vi "SettingsText.vi"(8 "Saved code":string, 10 "Python Code in":string, 11 "VI in":refnum<vi>) -> (2 "Python Code out":string, 3 "VI out":refnum<vi>)   [LabVIEW 2017]
panel:
  in  "Blob Params":T1={"Feature"=5, "Lab thresholds"="[10,90,-20,20,-20,20]", "Minimum Pixels"=100, "Minimum Area (box)"=100, "Merge"=TRUE, "Margin for merge"=10} {"Feature" items=["x", "y", "width", "height", "pixels", "cx", "cy", "rotation", "code", "count", "# blobs", "All parameters"]}
  in  "WiFi Info":T2
  in  "ROI":T3
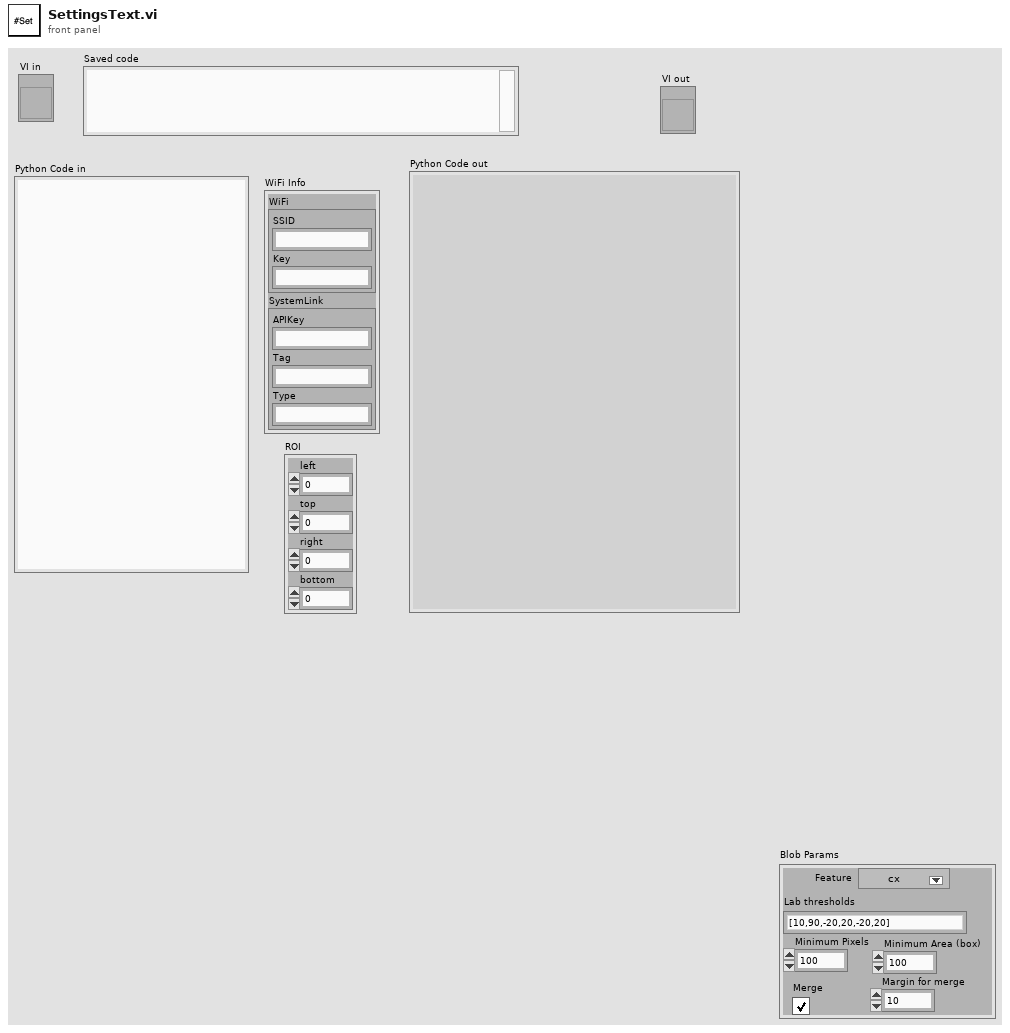
[diagram p1: front panel]
types:
  T1 = cluster{"Feature":u16, "Lab thresholds":string, "Minimum Pixels":i16, "Minimum Area (box)":i16, "Merge":bool, "Margin for merge":i16}
  T2 = cluster{"WiFi":cluster{"SSID":string, "Key":string}, "SystemLink":cluster{"APIKey":string, "Tag":string, "Type":string}}
  T3 = cluster{"left":i32, "top":i32, "right":i32, "bottom":i32}
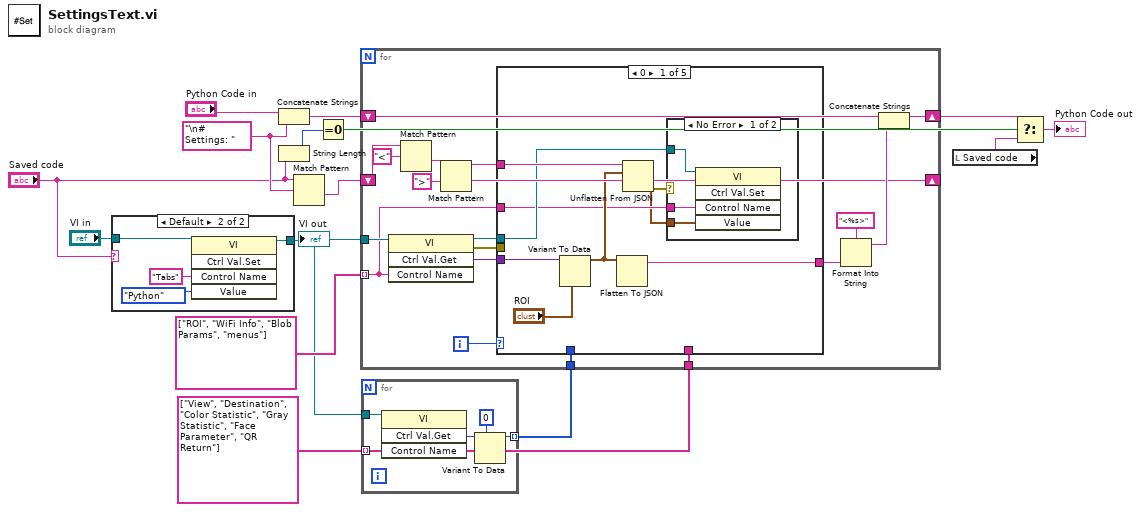
[diagram p0: block diagram]
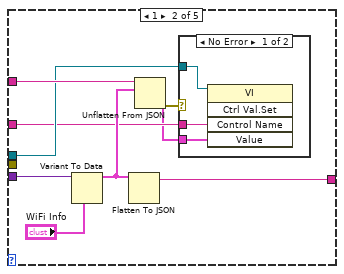
[diagram p4: hidden frame]
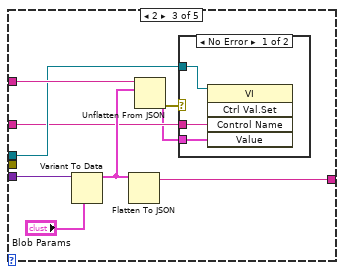
[diagram p6: hidden frame]
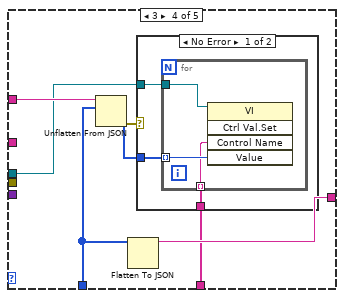
[diagram p8: hidden frame]
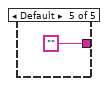
[diagram p10: hidden frame]
diagram:
  w9 = string[] ["View", "Destination", "Color Statistic", "Gray Statistic", "Face Parameter", "QR Return"]
  w11 = "\n# Settings: " ("string")
  n1 = case shown="Default" "Saved code" {
    tunnel: "VI in" -> [w16 w19]
    tunnel: [w16 w18] -> w2
    frame "\u0000" {
    }
    frame Default {
      n2 = invoke class="VI" method="Ctrl Val.Set"(reference=w19, "Control Name"="Tabs", "Value"=enum32{"Simple View", "REPL", "Python"}."Python" ("Tabs")) -> (reference out=w18:refnum<vi>)  [unwired: 2 in, 4 out]
    }
  }
  "VI out" <- w2
  n3 = Concatenate Strings("Python Code in", w11) -> (w13:string)
  n4 = String Length(string="Saved code") -> (length=w6:i32)
  n5 = Match Pattern(string="Saved code", regular expression=w11) -> (after substring=w10:string)  [unwired: 1 in, 3 out]
  n6 = Equal To 0?(x=w6) -> (x = 0?=w5:bool)
  n7 = for {
    tunnel: w2 -> [w25]
    tunnel: w9 -> [w24] mode=indexing
    tunnel: [w21] -> w12 mode=indexing
    n8 = invoke class="VI" method="Ctrl Val.Get"(reference=w25, "Control Name"=w24) -> ("Get Control Value Variant"=w23:variant)  [unwired: 2 in, 3 out]
    n9 = Variant To Data(type=0, Variant=w23) -> (data=w21:i32)  [unwired: 1 in, 1 out]
  }
  n10 = for {
    tunnel: w2 -> [w44]
    shift-right: [w38] -> w8
    shift-left: w13 -> [w39]
    tunnel: string[] ["ROI", "WiFi Info", "Blob Params", "menus"] -> [w28] mode=indexing
    tunnel: w12 -> [w35]
    shift-right: [w31] -> _
    shift-left: w10 -> [w26]
    tunnel: w9 -> [w27]
    i -> [w37]
    n11 = invoke class="VI" method="Ctrl Val.Get"(reference=w44, "Control Name"=w28) -> (reference out=w29:refnum<vi>, error out=w36:errorcluster, "Get Control Value Variant"=w43:variant)  [unwired: 2 in, 1 out]
    n12 = Match Pattern(string=w26, regular expression="<") -> (after substring=w33:string)  [unwired: 1 in, 3 out]
    n13 = Match Pattern(string=w33, regular expression=">") -> (before substring=w30:string, after substring=w31:string)  [unwired: 1 in, 2 out]
    n14 = case shown="0" w37 {
      tunnel: w43 -> [w53 w65 w77 _ _]
      tunnel: [w52 w64 w76 w87 "" ("JSON string")] -> w41
      tunnel: w36 -> [_ _ _ _ _]
      tunnel: w35 -> [_ _ _ w82 _]
      tunnel: w30 -> [w50 w63 w75 w86 _]
      tunnel: w29 -> [w47 w60 w72 w84 _]
      tunnel: w28 -> [w46 w59 w71 _ _]
      tunnel: w27 -> [_ _ _ w81 _]
      frame 0 {
        n15 = Variant To Data(type="ROI", Variant=w53) -> (data=w49:T3)  [unwired: 1 in, 1 out]
        n16 = Flatten To JSON(anything=w49) -> (JSON string=w52:string)  [unwired: 2 in, 1 out]
        n17 = Unflatten From JSON(JSON string=w50, type and defaults=w49) -> (value=w45:T3, error out=w48:errorcluster)  [unwired: 5 in]
        n18 = case shown="No Error" w48 {
          tunnel: w47 -> [w56 _]
          tunnel: w46 -> [w55 _]
          tunnel: w45 -> [w54 _]
          frame No Error {
            n19 = invoke class="VI" method="Ctrl Val.Set"(reference=w56, "Control Name"=w55, "Value"=w54) -> ()  [unwired: 2 in, 5 out]
          }
          frame Error {
          }
        }
      }
      frame 1 {
        n20 = Variant To Data(type="WiFi Info", Variant=w65) -> (data=w62:T2)  [unwired: 1 in, 1 out]
        n21 = Flatten To JSON(anything=w62) -> (JSON string=w64:string)  [unwired: 2 in, 1 out]
        n22 = Unflatten From JSON(JSON string=w63, type and defaults=w62) -> (value=w58:T2, error out=w61:errorcluster)  [unwired: 5 in]
        n23 = case shown="No Error" w61 {
          tunnel: w60 -> [w68 _]
          tunnel: w59 -> [w67 _]
          tunnel: w58 -> [w66 _]
          frame No Error {
            n24 = invoke class="VI" method="Ctrl Val.Set"(reference=w68, "Control Name"=w67, "Value"=w66) -> ()  [unwired: 2 in, 5 out]
          }
          frame Error {
          }
        }
      }
      frame 2 {
        n25 = Variant To Data(type="Blob Params", Variant=w77) -> (data=w74:T1)  [unwired: 1 in, 1 out]
        n26 = Flatten To JSON(anything=w74) -> (JSON string=w76:string)  [unwired: 2 in, 1 out]
        n27 = Unflatten From JSON(JSON string=w75, type and defaults=w74) -> (value=w70:T1, error out=w73:errorcluster)  [unwired: 5 in]
        n28 = case shown="No Error" w73 {
          tunnel: w72 -> [w80 _]
          tunnel: w71 -> [w79 _]
          tunnel: w70 -> [w78 _]
          frame No Error {
            n29 = invoke class="VI" method="Ctrl Val.Set"(reference=w80, "Control Name"=w79, "Value"=w78) -> ()  [unwired: 2 in, 5 out]
          }
          frame Error {
          }
        }
      }
      frame 3 {
        n30 = Unflatten From JSON(JSON string=w86, type and defaults=w82) -> (value=w83:i32[], error out=w85:errorcluster)  [unwired: 5 in]
        n31 = Flatten To JSON(anything=w82) -> (JSON string=w87:string)  [unwired: 2 in, 1 out]
        n32 = case shown="No Error" w85 {
          tunnel: w84 -> [w90 _]
          tunnel: w83 -> [w89 _]
          tunnel: w81 -> [w88 _]
          frame No Error {
            n33 = for {
              tunnel: w90 -> [w93]
              tunnel: w89 -> [w92] mode=indexing
              tunnel: w88 -> [w91] mode=indexing
              n34 = invoke class="VI" method="Ctrl Val.Set"(reference=w93, "Control Name"=w91, "Value"=w92) -> ()  [unwired: 2 in, 5 out]
            }
          }
          frame Error {
          }
        }
      }
      frame Default {
      }
    }
    n35 = Format Into String(format string="<%s>", w41) -> (resulting string=w40:string)  [unwired: 2 in, 1 out]
    n36 = Concatenate Strings(w39, w40) -> (w38:string)
  }
  n37 = local read "Saved code"() -> (w4:string)
  n38 = Select(t=w8, s=w5, f=w4) -> (s? t:f=→"Python Code out":string)
